vi "transmit.vi"(8 "error in (no error)":errorcluster, 11 "Modbus in":refnum<class "Modbus.lvclass">) -> (0 "error out":errorcluster, 3 "Modbus out":refnum<class "Modbus.lvclass">)   [LabVIEW 2015, in "RTModbus.lvlib" / "Modbus.lvclass"]
uses:
  Modbus.lvclass
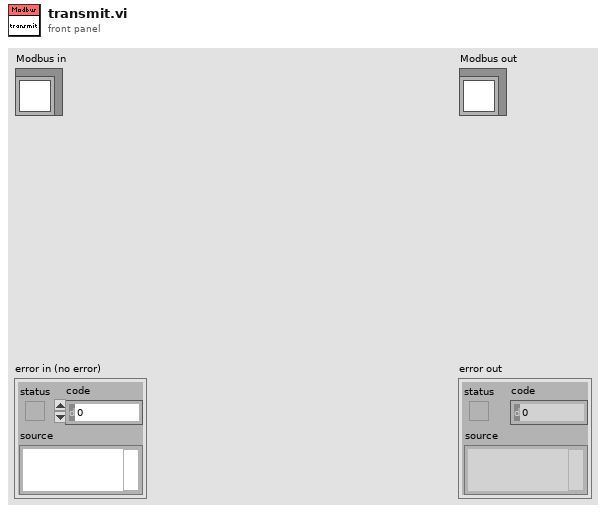
[diagram p1: front panel]
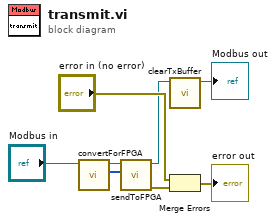
[diagram p0: block diagram]
diagram:
  n1 = call "convertForFPGA.vi"("Modbus in"="Modbus in") -> ("Data"=w3:u16[], "Modbus out"=w4:refnum<class "Modbus.lvclass">)  [unwired: 8 in, 1 out]
  n2 = call-dynamic "sendToFPGA.vi"("Data"=w3, "Modbus in"=w4) -> ("error out"=w8:errorcluster, "Modbus out"=w2:refnum<class "Modbus.lvclass">)  [unwired: 8 in]
  n3 = call "clearTxBuffer.vi"("Modbus in"=w2) -> ("Modbus out"=→"Modbus out":refnum<class "Modbus.lvclass">)  [unwired: 9 in, 1 out]
  n4 = Merge Errors("error in (no error)", w8) -> (→"error out":errorcluster)
